vi "HEWH Ritter Wet Meter Correction.vi"(7 "TC8-Gas Temp":dbl, 9 "volume (cuft)":dbl, 10 "flow (cuft/hr)":dbl, 11 "Data Cluster":T1) -> (0 "Corrected volume (cuft)":dbl, 1 "Corrected Volumetric Flow Rate (cuft/hr)":dbl, 2 "Volumetric Flow Rate (cuft/hr)":dbl, 3 "STP Correction Factor":dbl)   [LabVIEW 2020]
uses:
  Drivers/Alicat Gas Meter Driver/Sub-VIs/Data Cluster.ctl
panel:
  out "error out":errorcluster
  in  "error in":errorcluster
  # "Totalizer Timer"
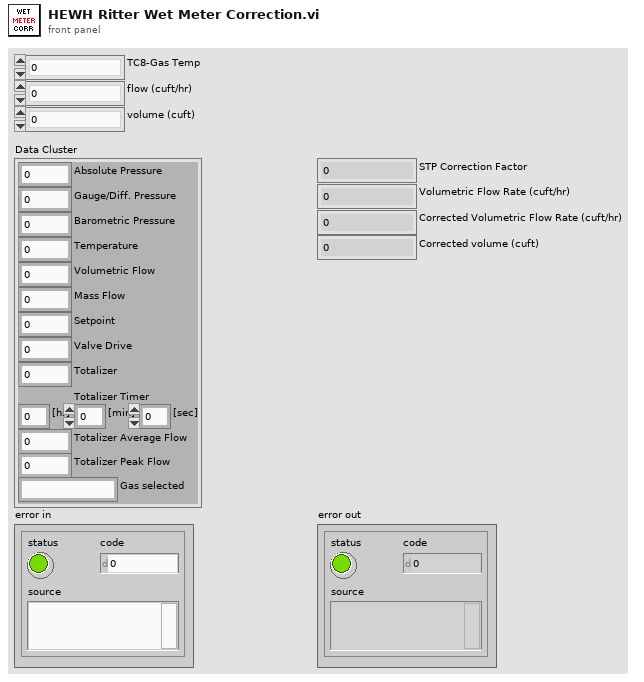
[diagram p1: front panel]
types:
  T1 = typedef "Data Cluster.ctl" = cluster{"Absolute Pressure":dbl, "Gauge/Diff. Pressure":dbl, "Barometric Pressure":dbl, "Temperature":dbl, "Volumetric Flow":dbl, "Mass Flow":dbl, "Setpoint":dbl, "Valve Drive":dbl, "Totalizer":dbl, "[hr]":dbl, "[min]":dbl, "[sec]":dbl, "Totalizer Average Flow":dbl, "Totalizer Peak Flow":dbl, "Gas selected":string}
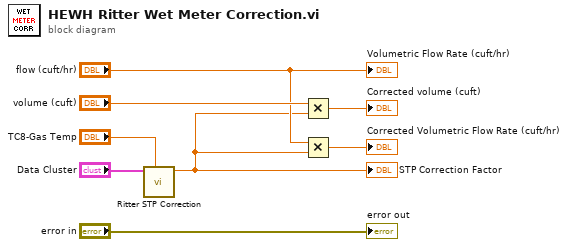
[diagram p0: block diagram]
diagram:
  n1 = call "Ritter STP Correction.vi"("TC8-Gas Temp"="TC8-Gas Temp", "Data Cluster"="Data Cluster") -> ("STP Correction Factor"=w3:dbl)  [unwired: 8 in, 1 out]
  "STP Correction Factor" <- w3
  n2 = Multiply(x="volume (cuft)", y=w3) -> (x*y=→"Corrected volume (cuft)":dbl)
  n3 = Multiply(x="flow (cuft/hr)", y=w3) -> (x*y=→"Corrected Volumetric Flow Rate (cuft/hr)":dbl)
  "error out" <- "error in"
  "Volumetric Flow Rate (cuft/hr)" <- "flow (cuft/hr)"
